vi "Register gRPC Methods.vi"(8 "error in (no error)":errorcluster, 11 "Template Server in":refnum<class "HVC6.lvclass">) -> (0 "error out":errorcluster, 3 "Template Server out":refnum<class "HVC6.lvclass">)   [LabVIEW 2019, in "HVC6.lvlib" / "HVC6.lvclass"]
uses:
  HVC6.lvclass
  typeDefs/Server Internal UEs.ctl
  typeDefs/Server Internal Message.ctl
  typeDefs/Server gRPC UEs.ctl
  gRPC lvSupport/Server API/typeDefs/gRPCId Cluster.ctl
  gRPC lvSupport/Server API/typeDefs/grpcId.ctl
  HVC6.lvclass/HVC6.ctl
  gRPC lvSupport/gprc-lvsupport.lvlib
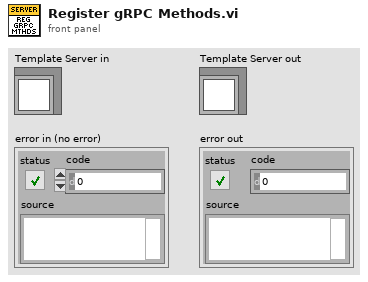
[diagram p1: front panel]
types:
  T1 = typedef "HVC6.lvlib/HVC6.lvclass/Server gRPC UEs.ctl" = cluster{"Invoke gRPC UE":refnum<user-event>, "Query gRPC UE":refnum<user-event>, "Register gRPC UE":refnum<user-event>, "OpenPWMSession gRPC UE":refnum<user-event>, "StartPWM gRPC UE":refnum<user-event>, "ModifyPWM gRPC UE":refnum<user-event>, "StopPWM gRPC UE":refnum<user-event>, "ClosePWMSession gRPC UE":refnum<user-event>}
  T2 = typedef "HVC6.lvlib/HVC6.lvclass/Server Internal UEs.ctl" = cluster{"Invoke Internal UE":refnum<user-event>, "Query Internal UE":refnum<user-event>, "Register Internal UE":refnum<user-event>, "OpenPWMSession Internal UE":refnum<user-event>, "StartPWM Internal UE":refnum<user-event>, "ModifyPWM Internal UE":refnum<user-event>, "StopPWM Internal UE":refnum<user-event>, "ClosePWMSession Internal UE":refnum<user-event>}
  T3 = typedef "HVC6.lvlib/gprc-lvsupport.lvlib/grpcId.ctl" = u64
  T4 = typedef "HVC6.lvlib/HVC6.lvclass/Server Internal Message UE.ctl" = refnum<user-event>
  T5 = typedef "HVC6.lvlib/gprc-lvsupport.lvlib/gRPCId Cluster UE.ctl" = refnum<user-event>
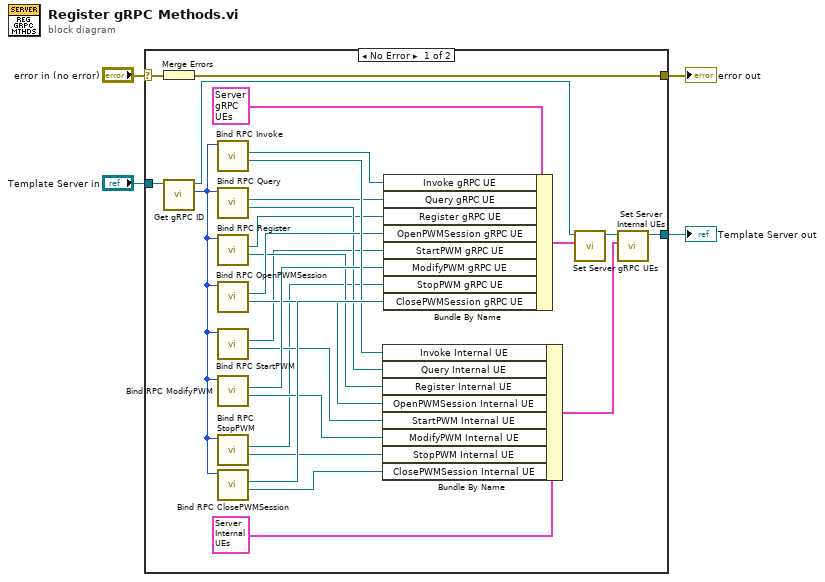
[diagram p0: block diagram]
diagram:
  n1 = case shown="No Error" "error in (no error)" {
    selector: "error in (no error)" -> [w22 w32]
    tunnel: "Template Server in" -> [w30 w33]
    tunnel: [w29 w32] -> w3
    tunnel: [w28 w33] -> w2
    frame No Error {
      n2 = Merge Errors(w22) -> (w29:errorcluster)
      n3 = call "Get gRPC ID.vi"("OOP Server in"=w30) -> ("gRPC ID"=w21:T3, "OOP Server out"=w31:refnum<class "HVC6.lvclass">)  [unwired: 9 in]
      n4 = call "Bind RPC Invoke.vi"("gRPCid server in"=w21) -> ("Invoke Internal UE"=w18:T4, "Invoke gRPC UE"=w17:T5)  [unwired: 7 in, 2 out]
      n5 = call "Bind RPC Query.vi"("gRPCid server in"=w21) -> ("Query Internal UE"=w12:T4, "Query gRPC UE"=w11:T5)  [unwired: 7 in, 2 out]
      n6 = call "Bind RPC Register.vi"("gRPCid server in"=w21) -> ("Register Internal UE"=w10:T4, "Register gRPC UE"=w9:T5)  [unwired: 7 in, 2 out]
      n7 = call "Bind RPC OpenPWMSession.vi"("gRPCid server in"=w21) -> ("OpenPWMSession Internal UE"=w14:T4, "OpenPWMSession gRPC UE"=w13:T5)  [unwired: 7 in, 2 out]
      n8 = call "Bind RPC StartPWM.vi"("gRPCid server in"=w21) -> ("StartPWM Internal UE"=w8:T4, "StartPWM gRPC UE"=w7:T5)  [unwired: 7 in, 2 out]
      n9 = call "Bind RPC ModifyPWM.vi"("gRPCid server in"=w21) -> ("ModifyPWM Internal UE"=w16:T4, "ModifyPWM gRPC UE"=w15:T5)  [unwired: 7 in, 2 out]
      n10 = call "Bind RPC StopPWM.vi"("gRPCid server in"=w21) -> ("StopPWM Internal UE"=w6:T4, "StopPWM gRPC UE"=w5:T5)  [unwired: 7 in, 2 out]
      n11 = call "Bind RPC ClosePWMSession.vi"("gRPCid server in"=w21) -> ("ClosePWMSession Internal UE"=w20:T4, "ClosePWMSession gRPC UE"=w19:T5)  [unwired: 7 in, 2 out]
      n12 = Bundle By Name ("Bundle Internal UEs")(cluster=T2 {"Invoke Internal UE"=refnum, "Query Internal UE"=refnum, "Register Internal UE"=refnum, "OpenPWMSession Internal UE"=refnum, "StartPWM Internal UE"=refnum, "ModifyPWM Internal UE"=refnum, "StopPWM Internal UE"=refnum, "ClosePWMSession Internal UE"=refnum} ("Server Internal UEs"), "Invoke Internal UE"=w18, "Query Internal UE"=w12, "Register Internal UE"=w10, "OpenPWMSession Internal UE"=w14, "StartPWM Internal UE"=w8, "ModifyPWM Internal UE"=w16, "StopPWM Internal UE"=w6, "ClosePWMSession Internal UE"=w20) -> (w27:T2)
      n13 = Bundle By Name ("Bundle gRPC UEs")(cluster=T1 {"Invoke gRPC UE"=refnum, "Query gRPC UE"=refnum, "Register gRPC UE"=refnum, "OpenPWMSession gRPC UE"=refnum, "StartPWM gRPC UE"=refnum, "ModifyPWM gRPC UE"=refnum, "StopPWM gRPC UE"=refnum, "ClosePWMSession gRPC UE"=refnum} ("gRPC Server Method Events"), "Invoke gRPC UE"=w17, "Query gRPC UE"=w11, "Register gRPC UE"=w9, "OpenPWMSession gRPC UE"=w13, "StartPWM gRPC UE"=w7, "ModifyPWM gRPC UE"=w15, "StopPWM gRPC UE"=w5, "ClosePWMSession gRPC UE"=w19) -> (w24:T1)
      n14 = call "Set Server gRPC UEs.vi"("Server gRPC UEs"=w24, "OOP Server in"=w31) -> ("OOP Server out"=w25:refnum<class "HVC6.lvclass">)  [unwired: 9 in]
      n15 = call "Set Server Internal UEs.vi"("Server Internal UEs"=w27, "OOP Server in"=w25) -> ("OOP Server out"=w28:refnum<class "HVC6.lvclass">)  [unwired: 9 in]
    }
    frame Error {
    }
  }
  "error out" <- w3
  "Template Server out" <- w2
